vi "CRYCreate data header string.vi"(0 "other delim":string, 1 "Data/Wave(if true=wave)?":bool, 3 "delimiter":enum16{"tab", "comma", "space", "other"}(ring), 4 "indices to save":i16[](array[numeric]), 5 "data series":string[](array[string])) -> (2 "export file header":string)   [LabVIEW 2013]
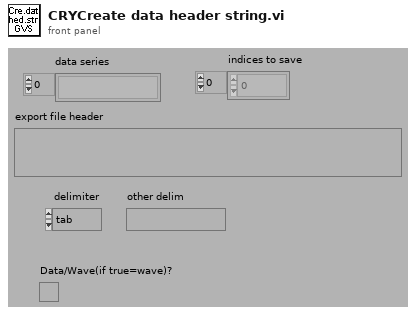
[diagram p1: front panel]
types:
  T1 = typedef "CRYData Cluster.ctl" = cluster{"Name":string, "Curve":cluster{"x":dbl, "y":dbl, "z":dbl}[], "X data":u16, "Y data":u16, "Z data":u16, "X axis":u16, "Y axis":u16, "Z axis":u16, "X unit":string, "Y unit":string, "Z unit":string, "X dB ref":dbl, "Y dB ref":dbl, "Z dB ref":dbl, "single val":bool, "protected":bool, "display X":bool, "display Y":bool, "display Z":bool, "Test Info":string, "Step No.":i32, "Plot Settings":cluster{"Color":u32, "Interpolation":u8, "Point Style":u8, "Line Style":u8, "Point Color":u32, "Line Width":u8, "Bar Plot Style":u8, "Fill To":i16}, "AutoProtect":bool}
  T2 = typedef "CRYWaveform Cluster.ctl" = cluster{"Waveform":cluster{"X0":dbl, "dX":dbl, "Y":sgl[]}, "X data":u16, "Y data":u16, "Y axis":u16, "X unit":string, "Y unit":string, "Y dB ref":dbl, "display Y":bool, "display X":bool, "Overload?":bool, "Test Info":string, "Step No.":i32, "Name":string, "protected":bool, "Sqc history":string[], "Signal Channel ID":i32, "Plot Settings":cluster{"Color":u32, "Interpolation":u8, "Point Style":u8, "Line Style":u8, "Point Color":u32, "Line Width":u8, "Bar Plot Style":u8, "Fill To":i16}, "AutoProtect":bool}
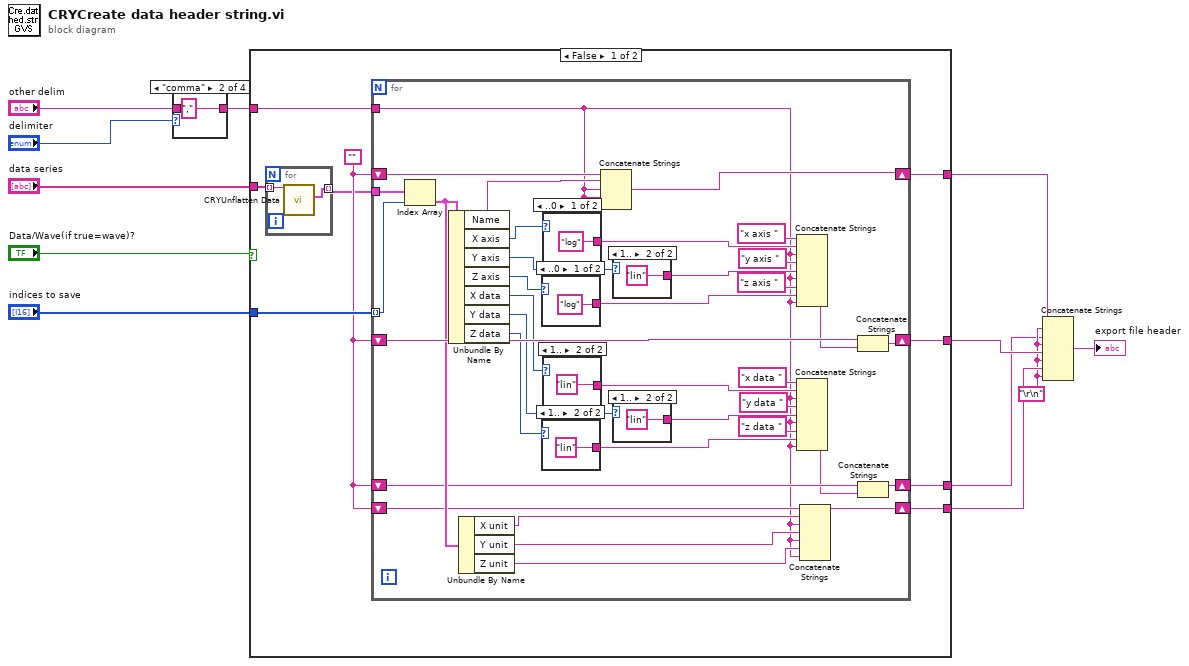
[diagram p0: block diagram]
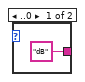
[diagram p2: hidden frame]
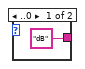
[diagram p3: hidden frame]
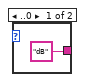
[diagram p4: hidden frame]
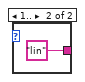
[diagram p5: hidden frame]
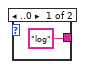
[diagram p6: hidden frame]
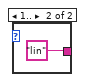
[diagram p7: hidden frame]
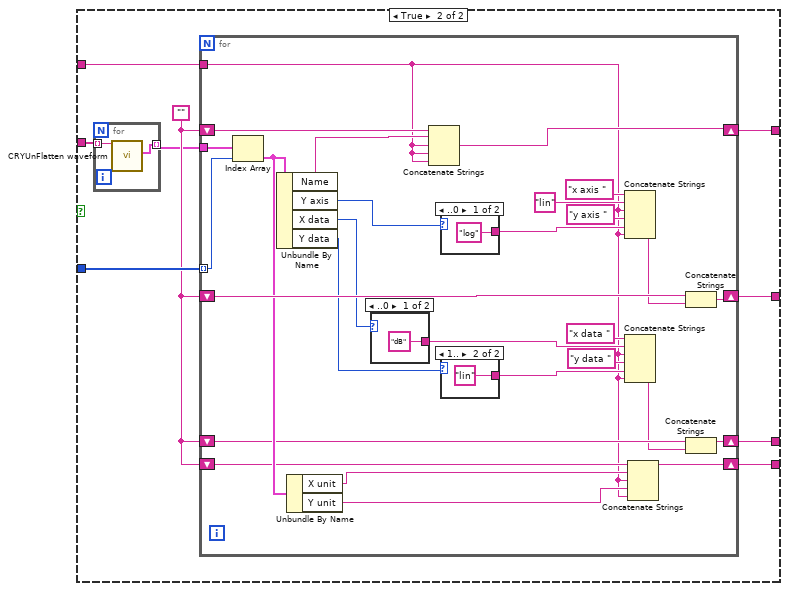
[diagram p8: hidden frame]
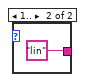
[diagram p9: hidden frame]
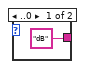
[diagram p10: hidden frame]
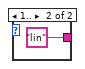
[diagram p11: hidden frame]
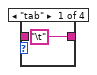
[diagram p12: hidden frame]
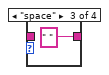
[diagram p13: hidden frame]
diagram:
  w7 = "\r\n"
  n1 = case shown="\"comma\"" "delimiter" {
    tunnel: "other delim" -> [_ _ _ w16]
    tunnel: ["\t" "," " " w16] -> w2
    frame "tab" {
    }
    frame "comma" {
    }
    frame "space" {
    }
    frame Default {
    }
  }
  n2 = case shown="False" "Data/Wave(if true=wave)?" {
    tunnel: "indices to save" -> [w25 w84]
    tunnel: [w24 w83] -> w11
    tunnel: [w23 w82] -> w10
    tunnel: [w21 w80] -> w8
    tunnel: [w20 w79] -> w6
    tunnel: "data series" -> [w18 w77]
    tunnel: w2 -> [w17 w76]
    frame False {
      w22 = ""
      n3 = for {
        tunnel: [w27] -> w19 mode=indexing
        tunnel: w18 -> [w26] mode=indexing
        n4 = call "CRYUnflatten Data.vi"("Unflatten data"=w26) -> ("Datum"=w27:T1)  [unwired: 8 in, 2 out]
      }
      n5 = for {
        tunnel: w19 -> [w63]
        tunnel: w25 -> [w62] mode=indexing
        shift-right: [w59] -> w21
        shift-left: w22 -> [w61]
        shift-right: [w47] -> w23
        shift-left: w22 -> [w49]
        shift-right: [w41] -> w24
        shift-left: w22 -> [w45]
        shift-right: [w32] -> w20
        shift-left: w22 -> [w34]
        tunnel: w17 -> [w28]
        n6 = Index Array(array=w63, index=w62) -> (element=w46:T1)
        n7 = Unbundle By Name(w46) -> ("Name"=w60:string, "X axis"=w58:u16, "Y axis"=w57:u16, "Z axis"=w56:u16, "X data"=w31:u16, "Y data"=w30:u16, "Z data"=w29:u16)
        n8 = Unbundle By Name(w46) -> ("X unit"=w44:string, "Y unit"=w43:string, "Z unit"=w42:string)
        n9 = case shown="..0" w56 {
          tunnel: ["log" "lin"] -> w50
          frame ..0 {
          }
          frame 1.. {
          }
        }
        n10 = case shown="1.." w29 {
          tunnel: ["dB" "lin"] -> w40
          frame ..0 {
          }
          frame 1.. {
          }
        }
        n11 = case shown="..0" w58 {
          tunnel: ["log" "lin"] -> w53
          frame ..0 {
          }
          frame 1.. {
          }
        }
        n12 = case shown="1.." w31 {
          tunnel: ["dB" "lin"] -> w37
          frame ..0 {
          }
          frame 1.. {
          }
        }
        n13 = Concatenate Strings(w61, w60, w28, w28, w28) -> (w59:string)
        n14 = case shown="1.." w57 {
          tunnel: ["log" "lin"] -> w52
          frame ..0 {
          }
          frame 1.. {
          }
        }
        n15 = case shown="1.." w30 {
          tunnel: ["dB" "lin"] -> w38
          frame ..0 {
          }
          frame 1.. {
          }
        }
        n16 = Concatenate Strings("x axis ", w53, w28, "y axis ", w52, w28, "z axis ", w50, w28) -> (w48:string)
        n17 = Concatenate Strings("x data ", w37, w28, "y data ", w38, w28, "z data ", w40, w28) -> (w33:string)
        n18 = Concatenate Strings(w45, w44, w28, w43, w28, w42, w28) -> (w41:string)
        n19 = Concatenate Strings(w49, w48) -> (w47:string)
        n20 = Concatenate Strings(w34, w33) -> (w32:string)
      }
    }
    frame True {
      w81 = ""
      n21 = for {
        tunnel: [w86] -> w78 mode=indexing
        tunnel: w77 -> [w85] mode=indexing
        n22 = call "CRYUnFlatten waveform.vi"("Unflatten Waveform"=w85) -> ("Waveform Cluster"=w86:T2)  [unwired: 8 in, 2 out]
      }
      n23 = for {
        tunnel: w78 -> [w114]
        tunnel: w84 -> [w113] mode=indexing
        shift-right: [w110] -> w80
        shift-left: w81 -> [w112]
        shift-right: [w102] -> w82
        shift-left: w81 -> [w104]
        shift-right: [w97] -> w83
        shift-left: w81 -> [w100]
        shift-right: [w90] -> w79
        shift-left: w81 -> [w92]
        tunnel: w76 -> [w87]
        n24 = Index Array(array=w114, index=w113) -> (element=w101:T2)
        n25 = Unbundle By Name(w101) -> ("Name"=w111:string, "Y axis"=w109:u16, "X data"=w89:u16, "Y data"=w88:u16)
        n26 = Unbundle By Name(w101) -> ("X unit"=w99:string, "Y unit"=w98:string)
        n27 = case shown="..0" w89 {
          tunnel: ["dB" "lin"] -> w95
          frame ..0 {
          }
          frame 1.. {
          }
        }
        n28 = Concatenate Strings(w112, w111, w87, w87, w87) -> (w110:string)
        n29 = case shown="..0" w109 {
          tunnel: ["log" "lin"] -> w105
          frame ..0 {
          }
          frame 1.. {
          }
        }
        n30 = case shown="1.." w88 {
          tunnel: ["dB" "lin"] -> w96
          frame ..0 {
          }
          frame 1.. {
          }
        }
        n31 = Concatenate Strings("x axis ", "lin", w87, "y axis ", w105, w87) -> (w103:string)
        n32 = Concatenate Strings("x data ", w95, w87, "y data ", w96, w87) -> (w91:string)
        n33 = Concatenate Strings(w100, w99, w87, w98, w87) -> (w97:string)
        n34 = Concatenate Strings(w104, w103) -> (w102:string)
        n35 = Concatenate Strings(w92, w91) -> (w90:string)
      }
    }
  }
  n36 = Concatenate Strings(w8, w7, w6, w7, w10, w7, w11, w7) -> (→"export file header":string)
